vi "AirHockey.vi"() -> ()   [LabVIEW 2017]
panel:
  out "Warning (C++)":string
  out "error out":errorcluster
  out "Frame":string
  in  "Sequence":string(combo)="Seq2m"
  out "OS Name":string
  out "computed command line":string
  out "standard error":string
  out "standard output":string
  in  "Pause":i32=5
  in  "Create Matlab Scoresheet":bool=TRUE
  in  "C1":u32(colorbox)=2298623
  in  "C0":u32(colorbox)=40718
  out "PNG picture":picture
  # "Projet 2018 - Air Hockey"
  # "WARNINGS &\nERRORS"
  # "© by M. Zemp, I. Scholl GM BA2"
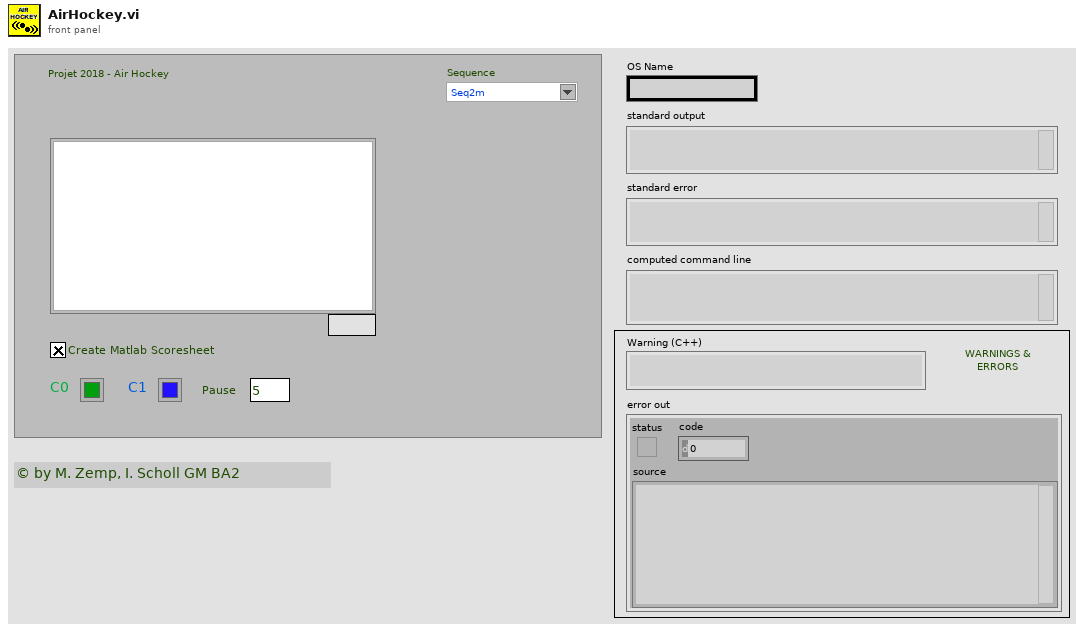
[diagram p1: front panel]
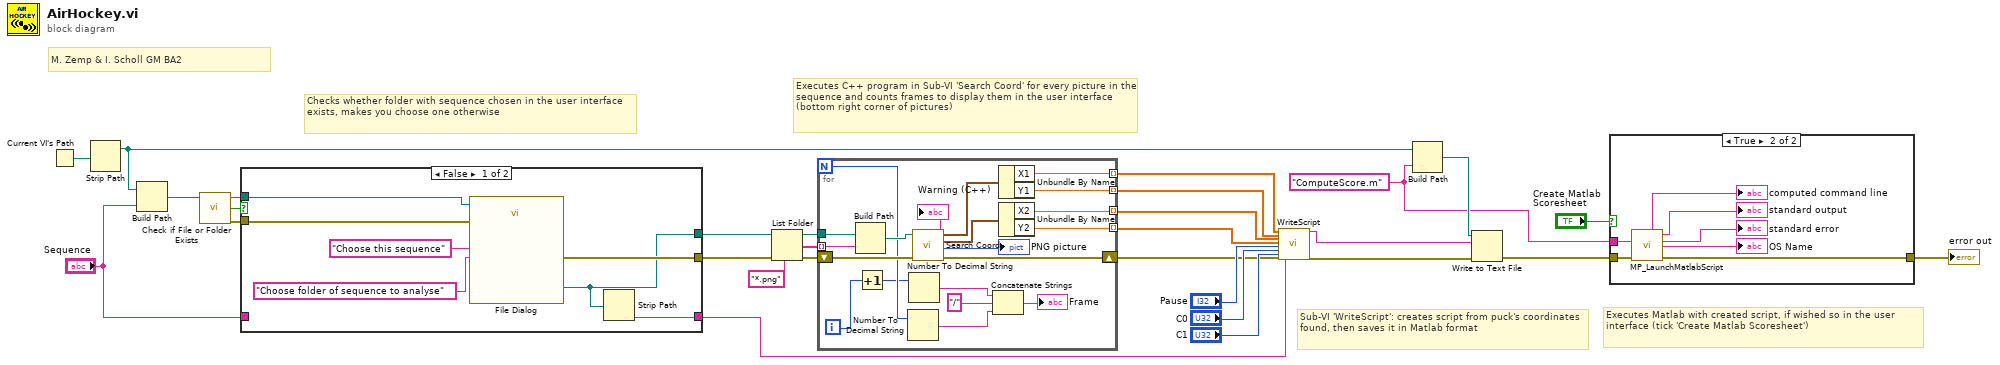
[diagram p0: block diagram]
diagram:
  w23 = "ComputeScore.m" ("name or relative path")
  # "M. Zemp & I. Scholl GM BA2"
  # "Executes Matlab with created script, if wished so in the user interface (tick 'Create Matlab Scoresheet')"
  # "Sub-VI 'WriteScript': creates script from puck's coordinates found, then saves it in Matlab format"
  # "Executes C++ program in Sub-VI 'Search Coord' for every picture in the sequence and counts frames to display them in the user interface (bottom right corner of pictures)"
  # "Checks whether folder with sequence chosen in the user interface exists, makes you choose one otherwise"
  n1 = Current VI's Path() -> (path=w29:path)
  n2 = Strip Path(path=w29) -> (stripped path=w28:path)  [unwired: 1 out]
  n3 = Build Path(base path=w28, name or relative path="Sequence") -> (appended path=w7:path)
  n4 = call <vilib>:"Check if File or Folder Exists.vi"("path"=w7) -> ("error out"=w25:errorcluster, "file or folder exists?"=w13:bool, "dup path"=w26:path)  [unwired: 8 in]
  n5 = case shown="False" w13 {
    tunnel: [w35 w38] -> w11
    tunnel: w26 -> [w34 w39]
    tunnel: w25 -> [w36 w38]
    tunnel: [w31 w39] -> w9
    tunnel: [w30 w37] -> w1
    tunnel: "Sequence" -> [_ w37]
    frame False {
      n6 = call "File Dialog"("start path"=w34, "prompt"="Choose folder of sequence to analyse" ("pattern label"), "button label"="Choose this sequence", "error in"=w36) -> ("selected path"=w31:path, "error out"=w35:errorcluster)  [unwired: 8 in, 2 out]
      n7 = Strip Path(path=w31) -> (name=w30:string)  [unwired: 1 out]
    }
    frame True {
    }
  }
  n8 = List Folder(path=w9, pattern="*.png", error in=w11) -> (path out=w6:path, filenames=w12:string[], error out=w10:errorcluster)  [unwired: 1 in, 1 out]
  n9 = for {
    N -> [w42]
    tunnel: w12 -> [w59] mode=indexing
    tunnel: w6 -> [w58]
    shift-right: [w55] -> w4
    shift-left: w10 -> [w56]
    tunnel: [w52] -> w18 mode=indexing
    tunnel: [w51] -> w17 mode=indexing
    tunnel: [w49] -> w16 mode=indexing
    tunnel: [w48] -> w15 mode=indexing
    i -> [w47]
    n10 = Build Path(base path=w58, name or relative path=w59) -> (appended path=w57:path)
    n11 = Increment(x=w47) -> (x+1=w41:i32)
    n12 = Number To Decimal String(number=w42) -> (decimal integer string=w44:string)  [unwired: 1 in]
    n13 = Number To Decimal String(number=w41) -> (decimal integer string=w46:string)  [unwired: 1 in]
    n14 = call "Search Coord.vi"("error in (no error)"=w56, "PNG Path"=w57) -> ("error out"=w55:errorcluster, "PNG picture"=→"PNG picture":picture, "Puck 2"=w50:cluster{"X2":dbl, "Y2":dbl}, "Puck 1"=w53:cluster{"X1":dbl, "Y1":dbl}, "Warning (C++)"=→"Warning (C++)":string)  [unwired: 5 in]
    n15 = Concatenate Strings(w46, "/", w44) -> (→"Frame":string)
    n16 = Unbundle By Name(w53) -> ("X1"=w52:dbl, "Y1"=w51:dbl)
    n17 = Unbundle By Name(w50) -> ("X2"=w49:dbl, "Y2"=w48:dbl)
  }
  n18 = call "WriteScript.vi"("X1"=w18, "Y1"=w17, "X2"=w16, "Y2"=w15, "Pause"="Pause", "C0"="C0", "C1"="C1", "error in"=w4, "Seq"=w1) -> ("concatenated string"=w19:string, "error out"=w3:errorcluster)  [unwired: 17 in]
  n19 = Build Path(base path=w28, name or relative path=w23) -> (appended path=w27:path)
  n20 = Write to Text File(file (use dialog)=w27, text=w19, error in=w3) -> (error out=w24:errorcluster)  [unwired: 1 in, 2 out]
  n21 = case shown="True" "Create Matlab Scoresheet" {
    tunnel: w24 -> [w60 w67]
    tunnel: w23 -> [_ w66]
    tunnel: [w60 w61] -> w14
    frame False {
    }
    frame True {
      n22 = call "MP_LaunchMatlabScript.vi"("error in (no error)"=w67, "matlab script name with extension"=w66) -> ("error out"=w61:errorcluster, "standard error"=→"standard error":string, "standard output"=→"standard output":string, "OS Name"=→"OS Name":string, "computed command line"=→"computed command line":string)  [unwired: 5 in]
    }
  }
  "error out" <- w14
